vi "MSR Sub.vi"(0 "MSR Fast Speed":dbl=1.0 min=-1.0 max=1.0, 1 "MSR Strafe Speed":dbl=1.0 min=-1.0 max=1.0, 2 "MSR Slow Speed":dbl=1.0 min=-1.0 max=1.0, 3 "MSR Fast Time":dbl=1.0 min=0.0, 4 "MSR Strafe Time":dbl=1.0 min=0.0, 5 "MSR Slow Time":dbl=1.0 min=0.0) -> ()   [LabVIEW 2017]
uses:
  <vilib>/Rock Robotics/Network Tables/NT Write Number.vi
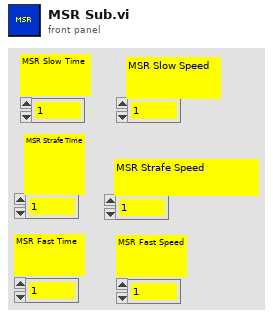
[diagram p1: front panel]
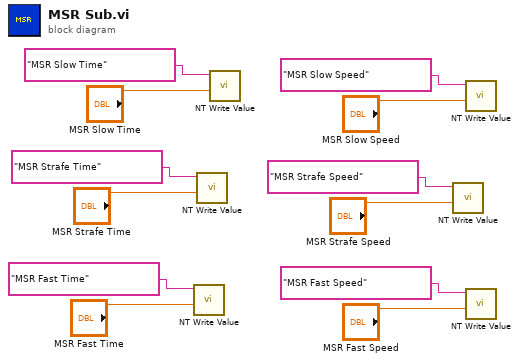
[diagram p0: block diagram]
diagram:
  n1 = call-poly <vilib>:"NT Write Value.vi"("Numeric"="MSR Fast Time", "Name"="MSR Fast Time") -> ()  [unwired: 9 in, 1 out]
  n2 = call-poly <vilib>:"NT Write Value.vi"("Numeric"="MSR Strafe Time", "Name"="MSR Strafe Time") -> ()  [unwired: 9 in, 1 out]
  n3 = call-poly <vilib>:"NT Write Value.vi"("Numeric"="MSR Slow Time", "Name"="MSR Slow Time") -> ()  [unwired: 9 in, 1 out]
  n4 = call-poly <vilib>:"NT Write Value.vi"("Numeric"="MSR Strafe Speed", "Name"="MSR Strafe Speed") -> ()  [unwired: 9 in, 1 out]
  n5 = call-poly <vilib>:"NT Write Value.vi"("Numeric"="MSR Slow Speed", "Name"="MSR Slow Speed") -> ()  [unwired: 9 in, 1 out]
  n6 = call-poly <vilib>:"NT Write Value.vi"("Numeric"="MSR Fast Speed", "Name"="MSR Fast Speed") -> ()  [unwired: 9 in, 1 out]
